vi "Get Scanner.vi"(8 "error in (no error)":errorcluster, 11 "Power Supply in":refnum<class "Power Supply.lvclass">) -> (0 "error out":errorcluster, 2 "Default Scanner out":refnum<class "Scanner.lvclass">)   [LabVIEW 2009, in "Power Supply.lvclass"]
doc: "(Dynamic) Returns the default Scanner object that scans over this Scannable. (Note that a Scannable may have multiple Scanners associated with it.) A Scanner is an analogue to an Iterator class in other languages."
uses:
  Power Supply.lvclass
  Scanners/Scanner/Scanner.lvclass
  Scanners/Magnetic Field/Magnetic Field.lvclass
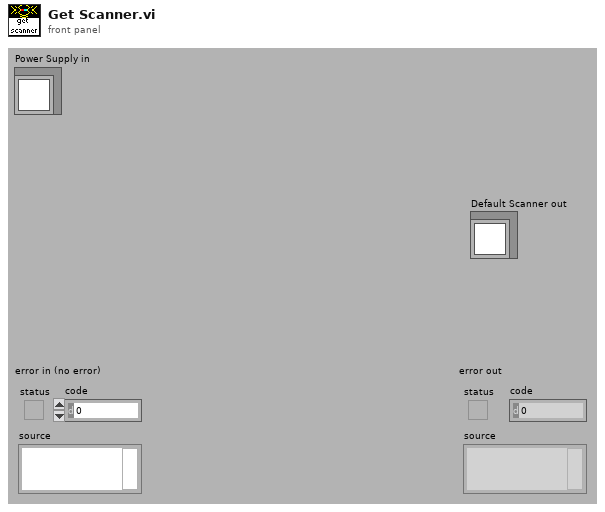
[diagram p1: front panel]
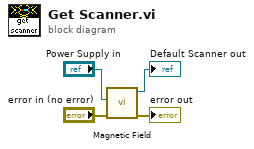
[diagram p0: block diagram]
diagram:
  n1 = call "Magnetic Field.vi"("error in (no error)"="error in (no error)", "Power Supply in"="Power Supply in") -> ("error out"=→"error out":errorcluster, "Magnetic Field.lvclass out"=→"Default Scanner out":refnum<class "Magnetic Field.lvclass">)  [unwired: 8 out]
